vi "DPOreadMeasurement.vi"(3 "错误输入（无错误）":errorcluster, 4 "通道":u8, 5 "VISA资源名称":refnum<visa-resource-name>) -> (0 "错误输出":errorcluster, 1 "data out":string, 2 "VISA资源名称输出":refnum<visa-resource-name>)   [LabVIEW 2012]
panel:
  out "结果字符串":string
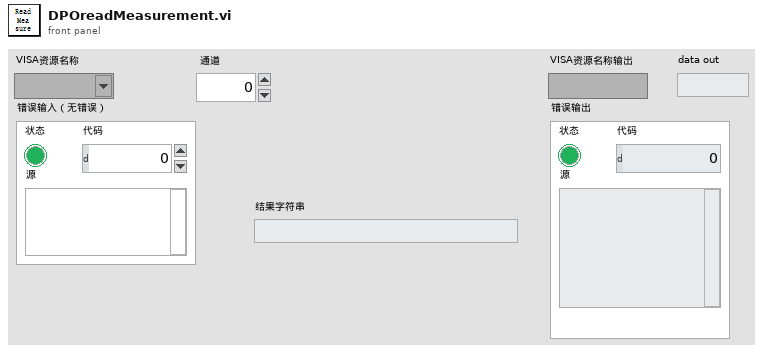
[diagram p1: front panel]
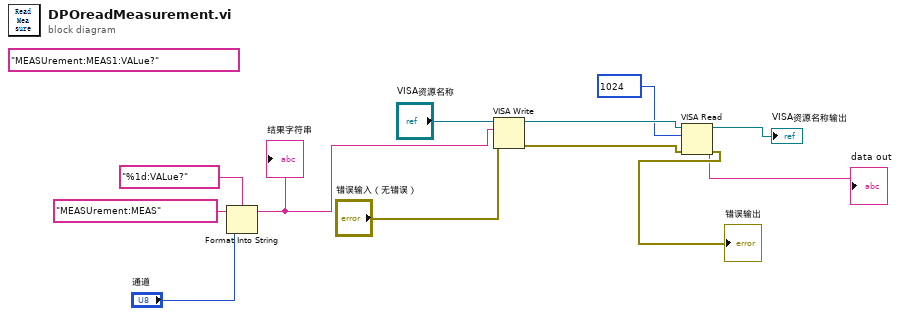
[diagram p0: block diagram]
diagram:
  (unwired) "MEASUrement:MEAS1:VALue?" ("写入缓冲区")
  n1 = Format Into String(format string="%1d:VALue?" ("格式字符串"), initial string="MEASUrement:MEAS" ("初始字符串"), "通道") -> (resulting string=w5:string)  [unwired: 1 in, 1 out]
  "结果字符串" <- w5
  n2 = VISA Write(VISA resource name="VISA资源名称", write buffer=w5, error in (no error)="错误输入（无错误）") -> (VISA resource name out=w10:refnum<visa-resource-name>, error out=w9:errorcluster)  [unwired: 1 out]
  n3 = VISA Read(VISA resource name=w10, byte count=u32 1024 ("字节总数"), error in (no error)=w9) -> (VISA resource name out=→"VISA资源名称输出":refnum<visa-resource-name>, read buffer=→"data out":string, error out=→"错误输出":errorcluster)  [unwired: 1 out]
